vi "Open_DB_Extract_Signals.vi"(0 "DBC  File Used":path) -> (2 "Refnum out":refnum<k21>)   [LabVIEW 2023]
uses:
  <resource>/objmgr/xnet.rc
panel:
  out "Array":T1(array[cluster])
  out "size(s)":i32
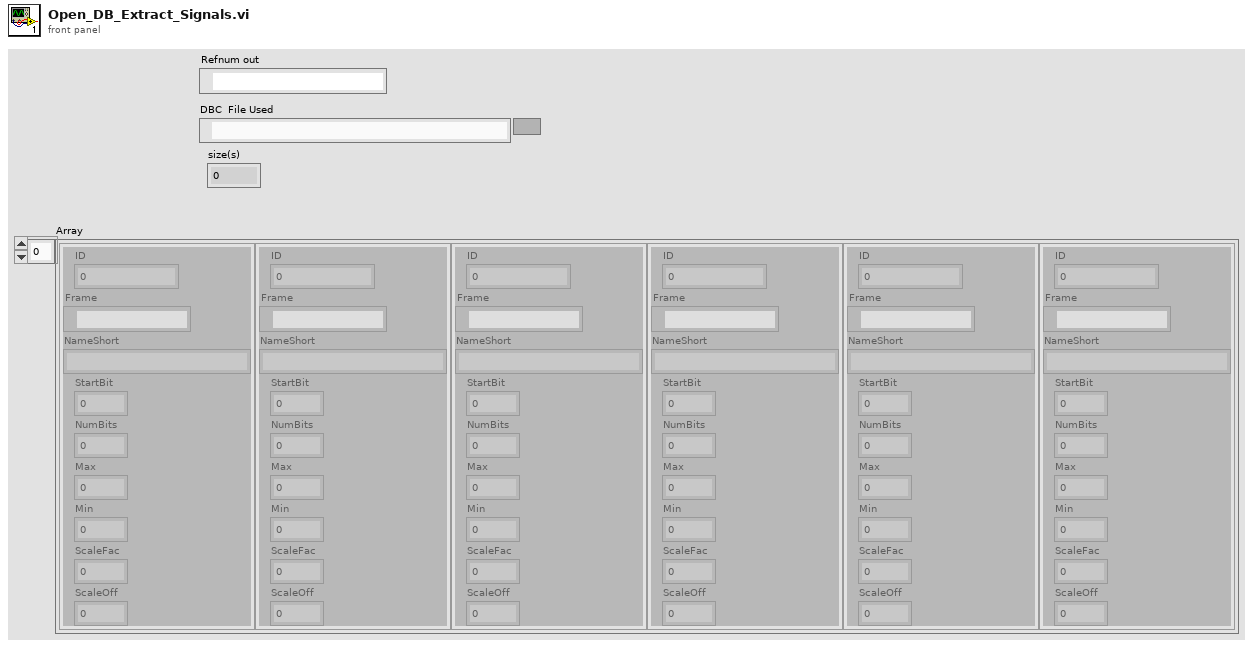
[diagram p1: front panel]
types:
  T1 = cluster{"ID":u32, "Frame":refnum<k21>, "NameShort":string, "StartBit":u32, "NumBits":u32, "Max":dbl, "Min":dbl, "ScaleFac":dbl, "ScaleOff":dbl}[]
  T2 = cluster{"ID":u32, "Frame":refnum<k21>, "NameShort":string, "StartBit":u32, "NumBits":u32, "Max":dbl, "Min":dbl, "ScaleFac":dbl, "ScaleOff":dbl}
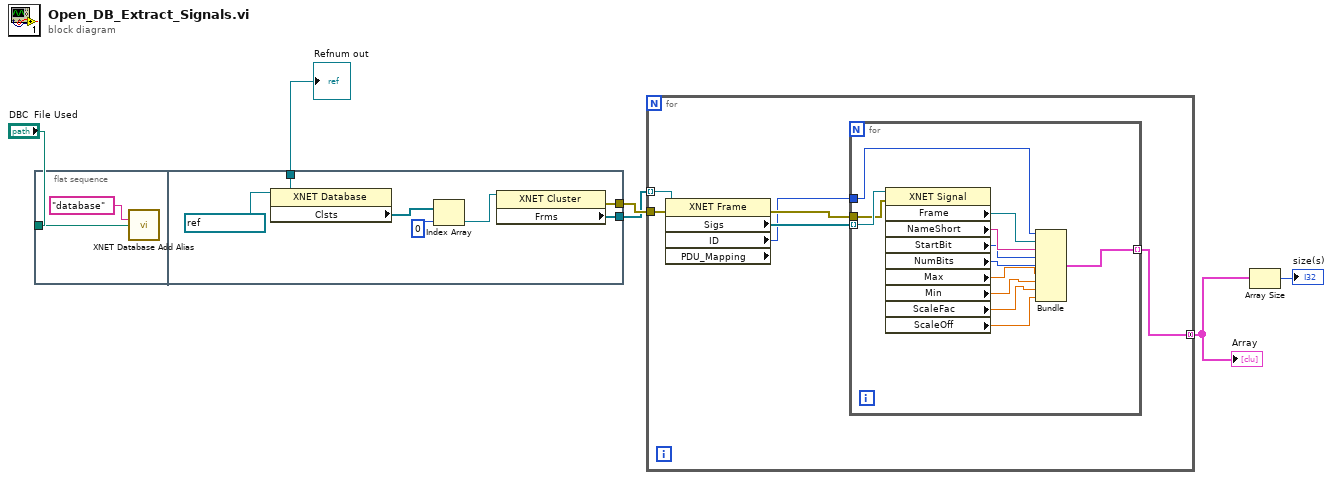
[diagram p0: block diagram]
diagram:
  n1 = flat-sequence {
    tunnel: "DBC  File Used" -> [w8]
    tunnel: [w11] -> w5
    tunnel: [w10] -> w4
    tunnel: [w9] -> w3
    frame #0 {
      n2 = call <vilib>:"XNET Database Add Alias.vi"("alias"="database", "filepath"=w8) -> ()  [unwired: 13 in, 1 out]
    }
    frame #1 {
      w11 = refnum<k21> "database" ("XNET Database")
      n3 = property class="XNET Database"(reference=w11) -> ("Clsts"=w14:refnum<k21>[])  [unwired: 1 in, 2 out]
      n4 = Index Array(array=w14, index=0) -> (element=w12:refnum<k21>)
      n5 = property class="XNET Cluster"(reference=w12) -> (error out=w10:errorcluster, "Frms"=w9:refnum<k21>[])  [unwired: 1 in, 1 out]
    }
  }
  n6 = for {
    tunnel: w4 -> [w20]
    tunnel: w3 -> [w17] mode=indexing
    tunnel: [w18] -> w2 mode=concatenating
    n7 = property class="XNET Frame" props=["Sigs", "ID", "PDU_Mapping"](reference=w17, error in=w20) -> (error out=w19:errorcluster, "Sigs"=w16:refnum<k21>[], "ID"=w15:u32)  [unwired: 2 out]
    n8 = for {
      tunnel: w16 -> [w32] mode=indexing
      tunnel: w19 -> [w31]
      tunnel: [w27] -> w18 mode=indexing
      tunnel: w15 -> [w22]
      n9 = property class="XNET Signal"(reference=w32, error in=w31) -> ("Frame"=w21:refnum<k21>, "NameShort"=w30:string, "StartBit"=w29:u32, "NumBits"=w28:u32, "Max"=w26:dbl, "Min"=w25:dbl, "ScaleFac"=w24:dbl, "ScaleOff"=w23:dbl)  [unwired: 2 out]
      n10 = Bundle("ID"=w22, "Frame"=w21, "NameShort"=w30, "StartBit"=w29, "NumBits"=w28, "Max"=w26, "Min"=w25, "ScaleFac"=w24, "ScaleOff"=w23) -> (w27:T2)  [unwired: 1 in]
    }
  }
  "Array" <- w2
  n11 = Array Size(array=w2) -> (size(s)=→"size(s)":i32)
  "Refnum out" <- w5
